vi "Read hostLoopPeriod_s.vi"(8 "error in (no error)":errorcluster, 11 "LoopConfig in":refnum<class "LoopConfig.lvclass">) -> (0 "error out":errorcluster, 2 "hostLoopPeriod_s":dbl=0.016, 3 "LoopConfig out":refnum<class "LoopConfig.lvclass">)   [LabVIEW 2013, in "ComponentData.lvlib" / "LoopConfig.lvclass"]
uses:
  <userlib>/Common/Component/common_application/RT/ComponentData/ConfigurationHandler/LoopConfig/LoopConfig.lvclass
  <userlib>/Common/Component/common_application/RT/ComponentData/ConfigurationHandler/LoopConfig/LoopConfig.lvclass/LoopConfig.ctl
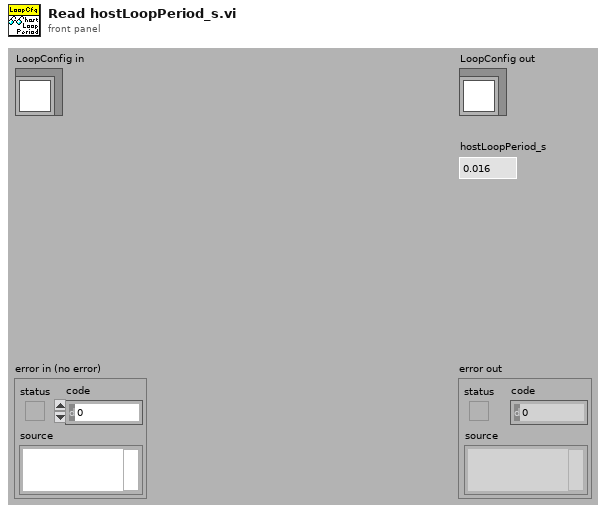
[diagram p1: front panel]
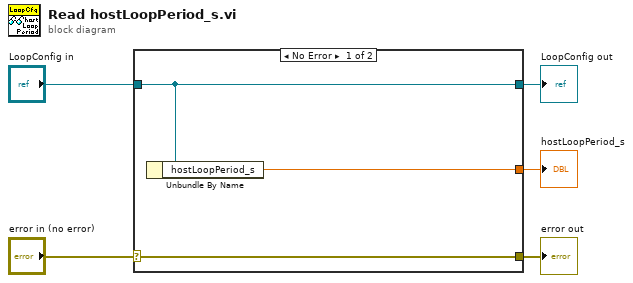
[diagram p0: block diagram]
diagram:
  n1 = case shown="No Error" "error in (no error)" {
    selector: "error in (no error)" -> [w8 w9]
    tunnel: [w8 w9] -> w4
    tunnel: [w7 w10] -> w2
    tunnel: "LoopConfig in" -> [w7 w10]
    tunnel: [w6 _] -> w1
    frame No Error {
      n2 = Unbundle By Name(w7) -> ("hostLoopPeriod_s"=w6:dbl)
    }
    frame Error {
    }
  }
  "error out" <- w4
  "LoopConfig out" <- w2
  "hostLoopPeriod_s" <- w1
